vi "Error Message.vi"(0 "VISA resource name":refnum<visa-resource-name>, 5 "Type of Dialog (1: OK Msg)":T1(ring)=enum."OK Message", 11 "error in (no error)":errorcluster {"code" format="%.0x"}) -> (3 "Status":bool, 4 "VISA resource name out":refnum<visa-resource-name>, 8 "Error Code (0)":i32, 10 "Error Message (empty)":string, 15 "error out":errorcluster {"code" format="%.0x"})   [LabVIEW 2010]
doc: "This VI contains all the intrument specific error codes and descriptions. Use this VI after executing several instrument driver VIs to recognize and display any errors that may have occurred."
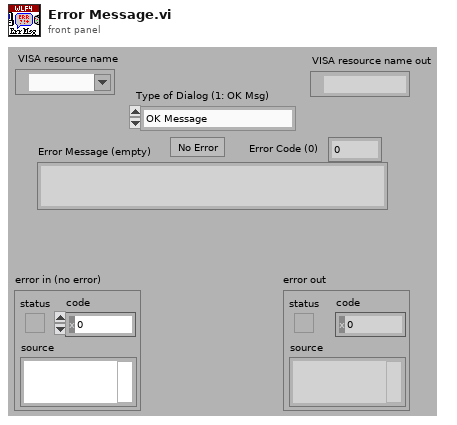
[diagram p1: front panel]
types:
  T1 = enum16{"No Dialog", "OK Message", "Continue or Stop Message"}
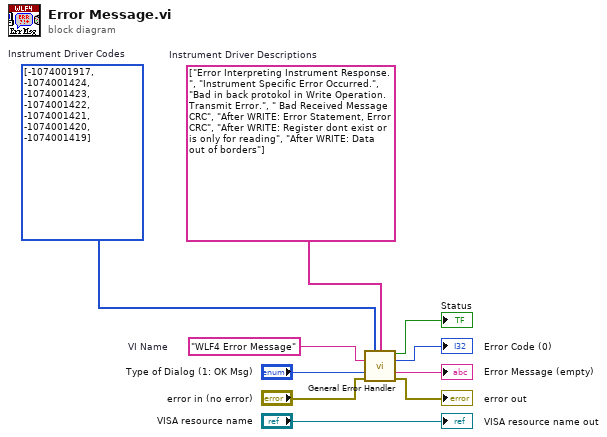
[diagram p0: block diagram]
diagram:
  w2 = i32[] [-1074001917, -1074001424, -1074001423, -1074001422, -1074001421, -1074001420, -1074001419]  # Instrument Driver Codes
  w1 = string[] ["Error Interpreting Instrument Response.", "Instrument Specific Error Occurred.", "Bad in back protokol in Write Operation. Transmit Error.", " Bad Received Message CRC", "After WRITE: Error Statement, Error CRC", "After WRITE: Register dont exist or is only for reading", "After WRITE: Data out of borders"]  # Instrument Driver Descriptions
  w7 = "WLF4 Error Message"  # VI Name
  n1 = call <vilib>:"General Error Handler.vi"("[user-defined codes]"=w2, "[user-defined descriptions]"=w1, "[error source] (\" \")"=w7, "type of dialog (OK msg:1)"="Type of Dialog (1: OK Msg)", "error in (no error)"="error in (no error)") -> ("error?"=→"Status":bool, "code out"=→"Error Code (0)":i32, "message"=→"Error Message (empty)":string, "error out"=→"error out":errorcluster)  [unwired: 6 in, 1 out]
  "VISA resource name out" <- "VISA resource name"
